vi "Spectrograph_putSample_loopTime.vi"(8 "error in (no error)":errorcluster, 11 "loopTime_Ctl":T1) -> (0 "error out":errorcluster, 2 "function return":i32, 3 "loopTime_Ctl out":T1)   [LabVIEW 2016, in "SALLV_Spectrograph.lvlib"]
doc: "int Spectrograph_shm_putSample_loopTimeLV(Spectrograph_loopTimeLV *loopTime_Ctl );"
uses:
  SALLV_Spectrograph.lvlib
  DataTypes/loopTime.ctl
  SALLV_Spectrograph.so
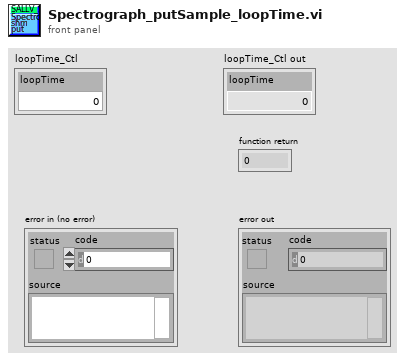
[diagram p1: front panel]
types:
  T1 = typedef "SALLV_Spectrograph.lvlib/loopTime.ctl" = cluster{"loopTime":dbl}
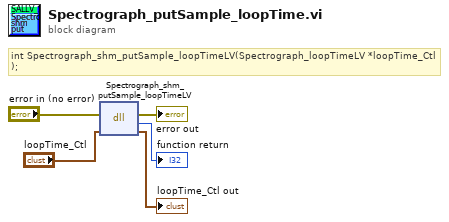
[diagram p0: block diagram]
diagram:
  # "int Spectrograph_shm_putSample_loopTimeLV(Spectrograph_loopTimeLV *loopTime_Ctl );"
  n1 = dll-call lib="home/harini/TCS/SALLV_Spectrograph/SALLV_Spectrograph.*" fn="Spectrograph_shm_putSample_loopTimeLV"(error in="error in (no error)", "loopTime_Ctl"="loopTime_Ctl") -> (error out=→"error out":errorcluster, →"function return":i32, "loopTime_Ctl"=→"loopTime_Ctl out":T1)  [unwired: 2 in, 1 out]
